vi "Clean Up Actor.vi"(8 "error in (no error)":errorcluster, 11 "Car Wash Console in":refnum<class "Car Wash Console.lvclass">) -> (0 "error out":errorcluster, 3 "Car Wash Console out":refnum<class "Car Wash Console.lvclass">)   [LabVIEW 2016, in "CLD Exam - Car Wash.lvlib" / "Car Wash Console.lvclass"]
doc: "--\nCopyright © 2017 Composed SystemsI All rights reserved.\n\nAuthor: Jon McBee <jon.mcbee@composed.io>\n\nThis library is provided \"AS IS\" ,WITHOUT WARRANTIES OR\nCONDITIONS OF ANY KIND, either express or implied.\n\nComposed Systems -- composed.io\n\nStream 0.0.1.1\nJon McBee - Composed Systems\nCopyright (c) 2017, Composed Systems"
uses:
  Car Wash Console.lvclass
  D:/Repos/Stream/software/Mediator/Classes/Mediated Actor/Mediated Actor.lvclass
  Mediator/Classes/Message Broker Interface/Message Broker Interface.lvclass
  Mediator/Classes/Mediated Synchronous Actor/Mediated Synchronous Actor.lvclass
  Mediator/Classes/Mediated Actor/Mediated Actor.lvclass
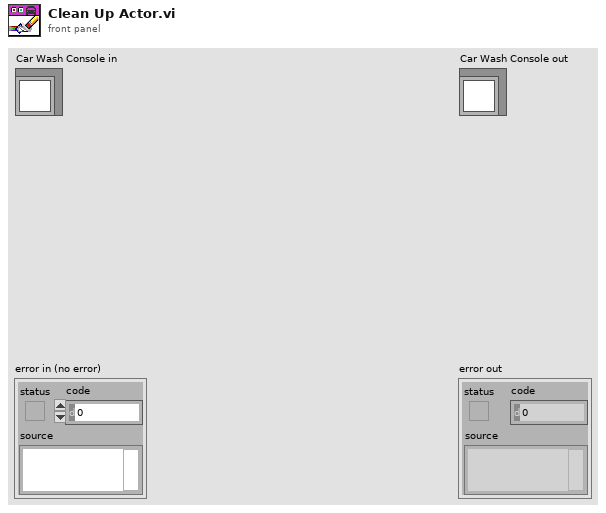
[diagram p1: front panel]
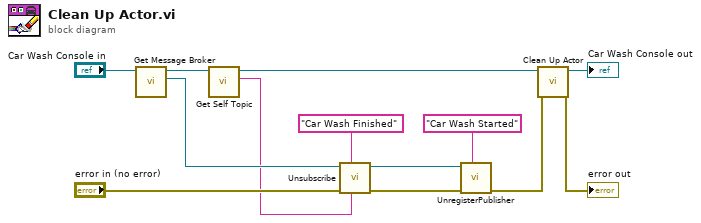
[diagram p0: block diagram]
diagram:
  n1 = call "Get Message Broker.vi"("Mediated Actor in"="Car Wash Console in") -> ("Message Broker"=w5:refnum<class "Message Broker Interface.lvclass">, "Mediated Actor out"=w10:refnum<class "Car Wash Console.lvclass">)  [unwired: 9 in]
  n2 = call "Get Self Topic.vi"("Mediated Actor in"=w10) -> ("Topic.Self"=w3:string, "Mediated Actor out"=w9:refnum<class "Car Wash Console.lvclass">)  [unwired: 9 in]
  n3 = call-dynamic "Unsubscribe.vi"("Subscriber Name"=w3, "Topic Name"="Car Wash Finished", "error in (no error)"="error in (no error)", "Message Broker Interface in"=w5) -> ("error out"=w6:errorcluster, "Message Broker Interface out"=w4:refnum<class "Message Broker Interface.lvclass">)  [unwired: 6 in]
  n4 = call-dynamic "UnregisterPublisher.vi"("Topic Name"="Car Wash Started", "error in (no error)"=w6, "Message Broker Interface in"=w4) -> ("error out"=w8:errorcluster)  [unwired: 7 in, 1 out]
  n5 = call-parent "Clean Up Actor.vi"("error in (no error)"=w8, "Mediated Actor in"=w9) -> ("error out"=→"error out":errorcluster, "Mediated Actor out"=→"Car Wash Console out":refnum<class "Car Wash Console.lvclass">)  [unwired: 8 in]
